vi "DAQmx Create DO Channel (sub).vi"(0 "task in":refnum<k21>, 1 "virtual channel name":string, 2 "line grouping":i32(ring) items=["one channel for each line", "one channel for all lines"], 5 "physical channel name":tag, 7 "measurement type":i32(ring)=10421 items=["digital output"=10421], 11 "error in":errorcluster) -> (4 "task out":refnum<k21>, 6 "channel names":string, 15 "error out":errorcluster)   [LabVIEW 2013]
uses:
  nilvaiu.dll
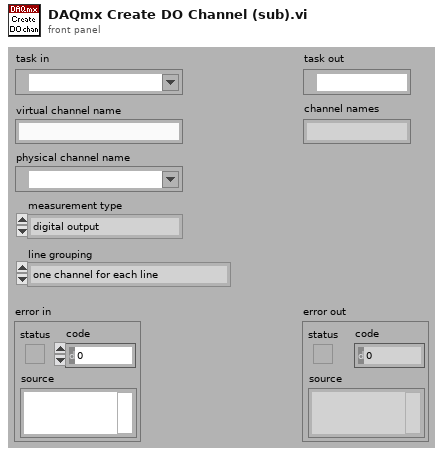
[diagram p1: front panel]
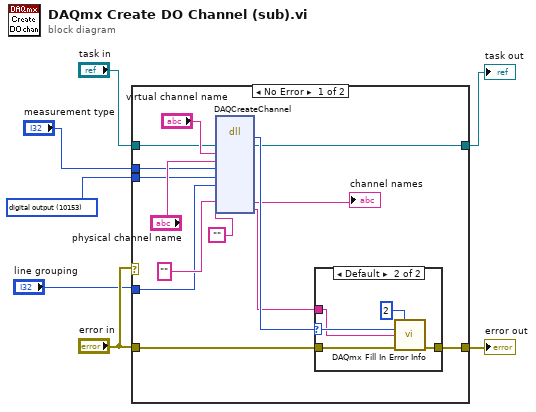
[diagram p0: block diagram]
diagram:
  w4 = 10153 items=["analog input"=10100, "analog output"=10102, "digital input"=10151, "digital output"=10153, "counter input"=10131, "counter output"=10132] ("channel type")
  n1 = case shown="No Error" "error in" {
    tunnel: [w17 w29] -> w7
    tunnel: "error in" -> [w19 w29]
    tunnel: "task in" -> [w8 w28]
    tunnel: "measurement type" -> [w16 _]
    tunnel: w4 -> [w15 _]
    tunnel: "line grouping" -> [w13 _]
    tunnel: [w9 w28] -> w1
    frame No Error {
      n2 = dll-call lib="nilvaiu.*" fn="DAQCreateChannel"("taskID"=w8, "virtual chnanel name"="virtual channel name", "physical channel name"="physical channel name", "measurement type"=w16, "channel type"=w15, "line grouping"=w13, "customScale"="", "channel names"="" ("custom scale")) -> (w18:i32, "taskID"=w9:refnum<k21>, "channel names"=→"channel names":string, "extendedErrorIndo"=w11:string)  [unwired: 8 in, 4 out]
      n3 = case shown="Default" w18 {
        selector: w18 -> [_ w25]
        tunnel: w19 -> [w22 w27]
        tunnel: [w22 w26] -> w17
        tunnel: w11 -> [_ w24]
        frame 0 {
        }
        frame Default {
          n4 = call "DAQmx Fill In Error Info.vi"("depth"=2, "status code"=w25, "extended error info"=w24, "error in"=w27) -> ("error out"=w26:errorcluster)  [unwired: 1 in, 10 out]
        }
      }
    }
    frame Error {
    }
  }
  "error out" <- w7
  "task out" <- w1
